vi "Set Disabled.vi"(8 "error in (no error)":errorcluster, 10 "Disabled":bool, 11 "DblStatusIndicator in":refnum<class "DblStatusIndicator.lvclass">) -> (0 "error out":errorcluster, 3 "DblStatusIndicator out":refnum<class "DblStatusIndicator.lvclass">)   [LabVIEW 2020, in "VolatusGUIElements.lvlib" / "DblStatusIndicator.lvclass"]
uses:
  DblStatusIndicator.lvclass
  DblStatusIndicator.lvclass/DblStatusIndicator.ctl
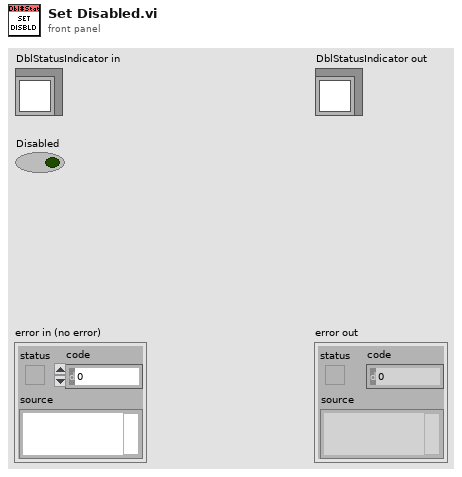
[diagram p1: front panel]
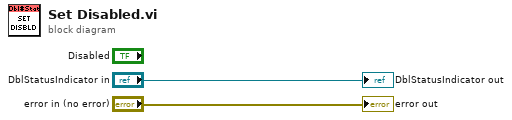
[diagram p0: block diagram]
diagram:
  "error out" <- "error in (no error)"
  "DblStatusIndicator out" <- "DblStatusIndicator in"
